vi "BaseProvider_DesignPattern_GetPatterns.vi"(1 "FilterOnProviders(Ignored If Empty)":string, 2 "FilterOnTemplate(Ignored If Empty)":string, 5 "error in (no error)":errorcluster) -> (15 "DesignPatterns":T1[](array[typedef]), 19 "error out":errorcluster)   [LabVIEW 2016]
uses:
  <resource>/Framework/Providers/Open_GDS/ClassProviders/Provider_BaseClassInterface/DesignPatternsData.ctl
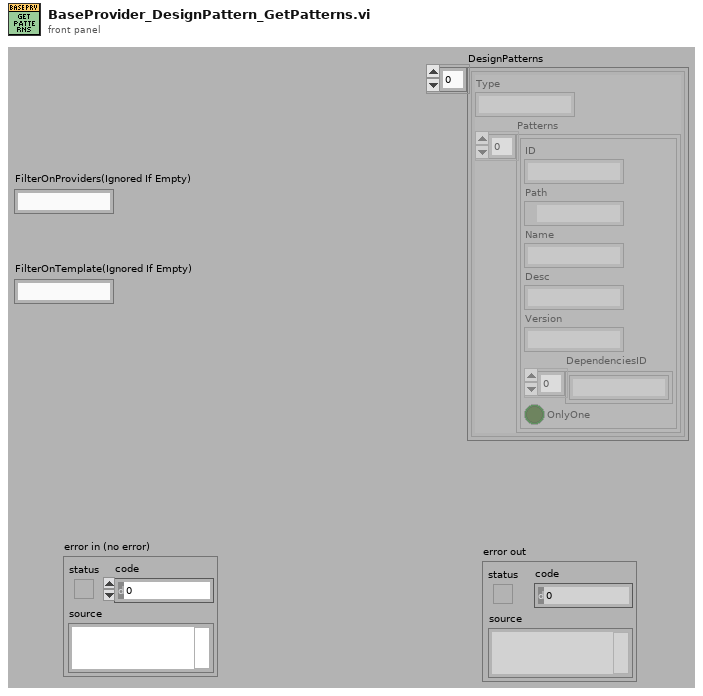
[diagram p1: front panel]
types:
  T1 = typedef "DesignPatternsData.ctl" = cluster{"Type":string, "Patterns":cluster{"ID":string, "Path":path, "Name":string, "Desc":string, "Version":string, "DependenciesID":string[], "OnlyOne":bool}[]}
  T2 = cluster{"Cancelled":bool, "IniFiles":path[], "IniFilesContent":cluster{"ID":string, "Version":string, "PlugIn":path, "Type":string, "Name":string, "Desc":string, "Supports":cluster{"Provider":string, "Templates":string}[], "DependenciesID":string[], "OnlyOne":bool}[], "DesignPatterns":T1[]}
  T3 = cluster{"ID":string, "Version":string, "PlugIn":path, "Type":string, "Name":string, "Desc":string, "Supports":cluster{"Provider":string, "Templates":string}[], "DependenciesID":string[], "OnlyOne":bool}[]
  T4 = cluster{"ID":string, "Version":string, "PlugIn":path, "Type":string, "Name":string, "Desc":string, "Supports":cluster{"Provider":string, "Templates":string}[], "DependenciesID":string[], "OnlyOne":bool}
  T5 = cluster{"ID":string, "Path":path, "Name":string, "Desc":string, "Version":string, "DependenciesID":string[], "OnlyOne":bool}[]
  T6 = cluster{"ID":string, "Path":path, "Name":string, "Desc":string, "Version":string, "DependenciesID":string[], "OnlyOne":bool}
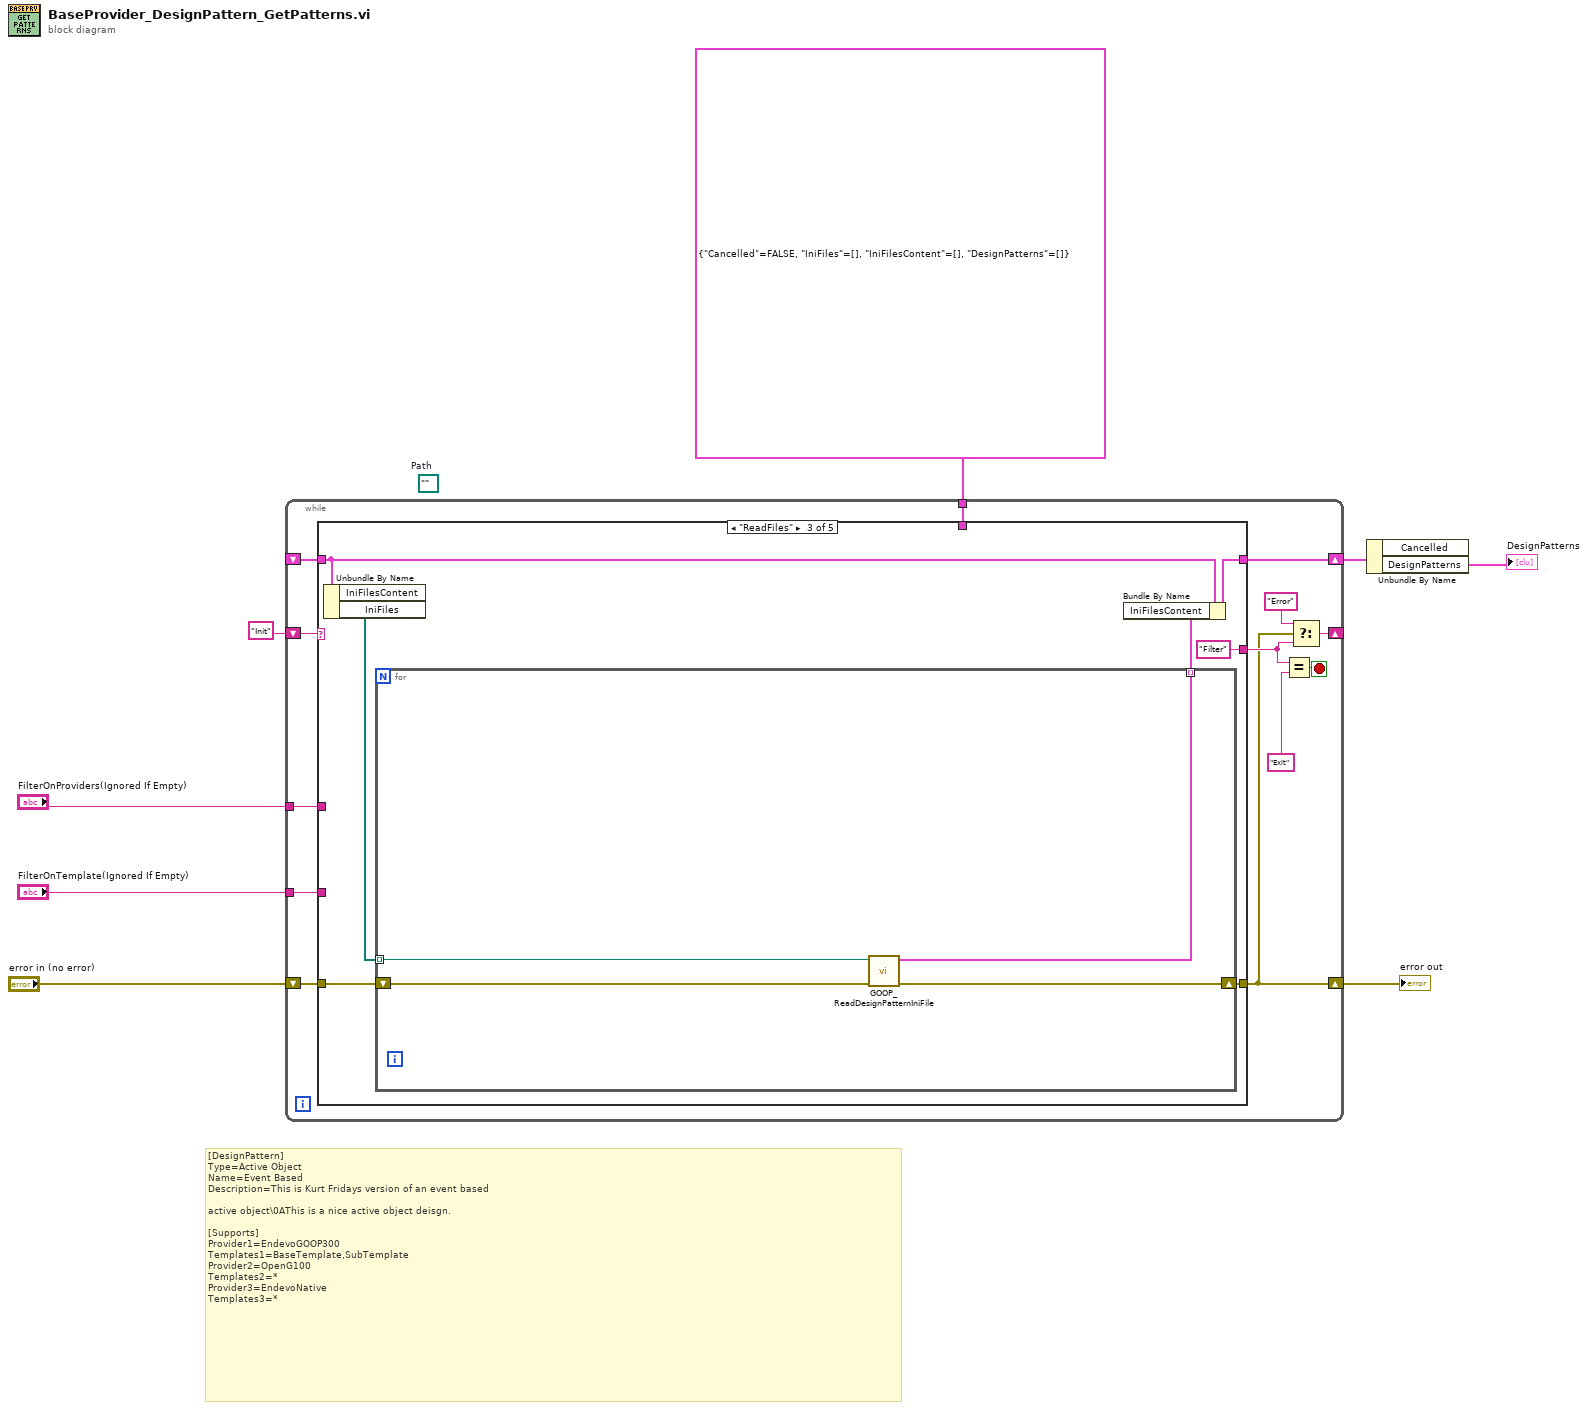
[diagram p0: block diagram]
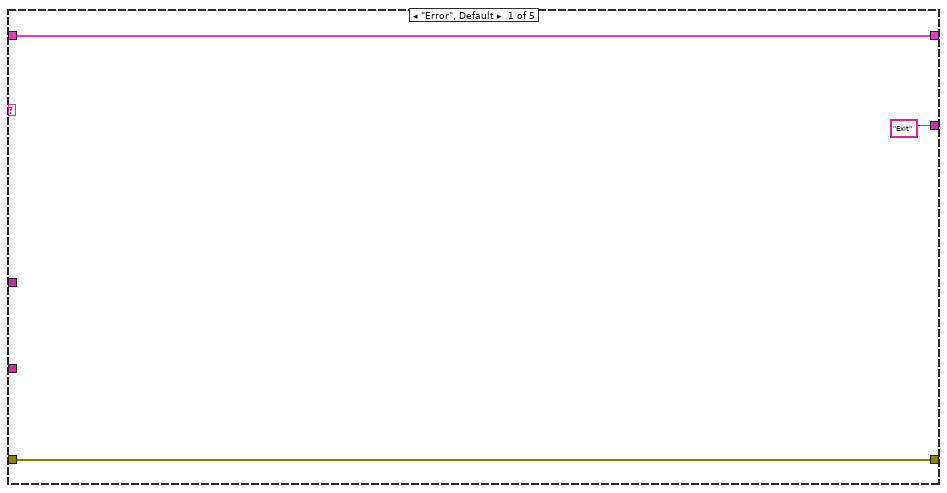
[diagram p2: hidden frame]
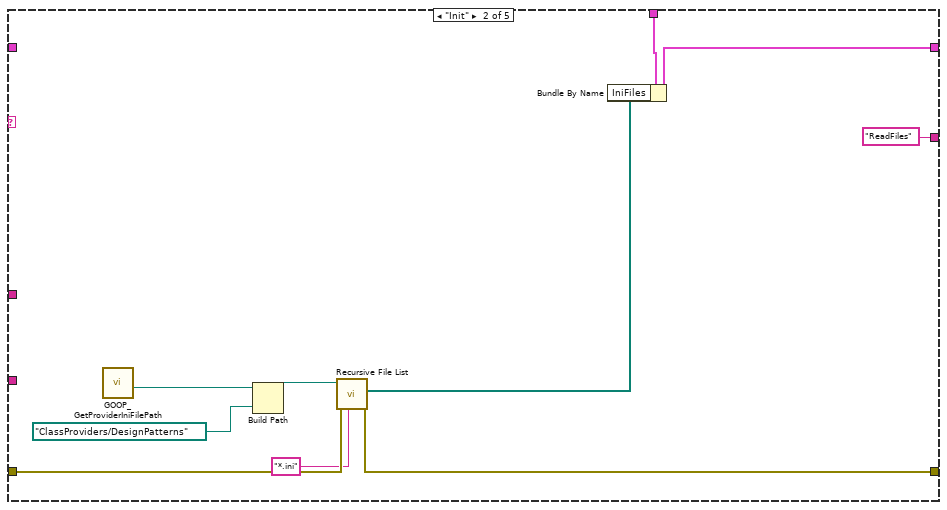
[diagram p3: hidden frame]
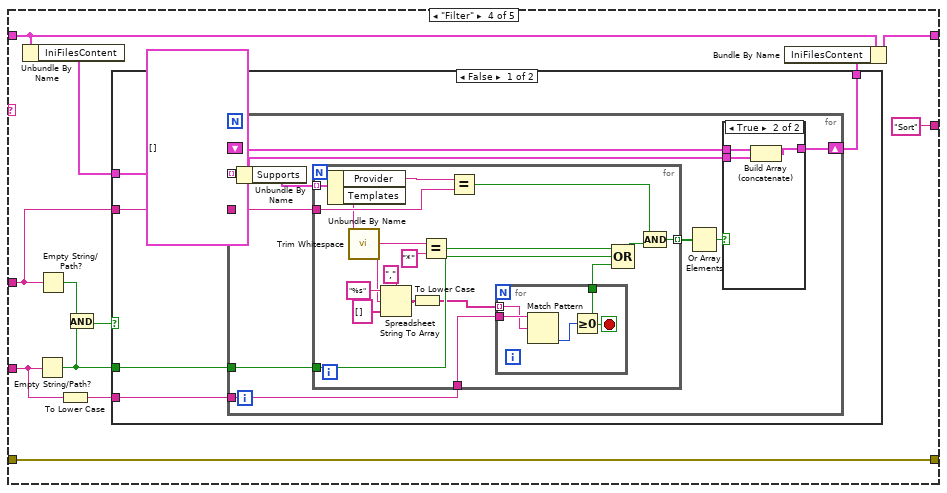
[diagram p4: hidden frame]
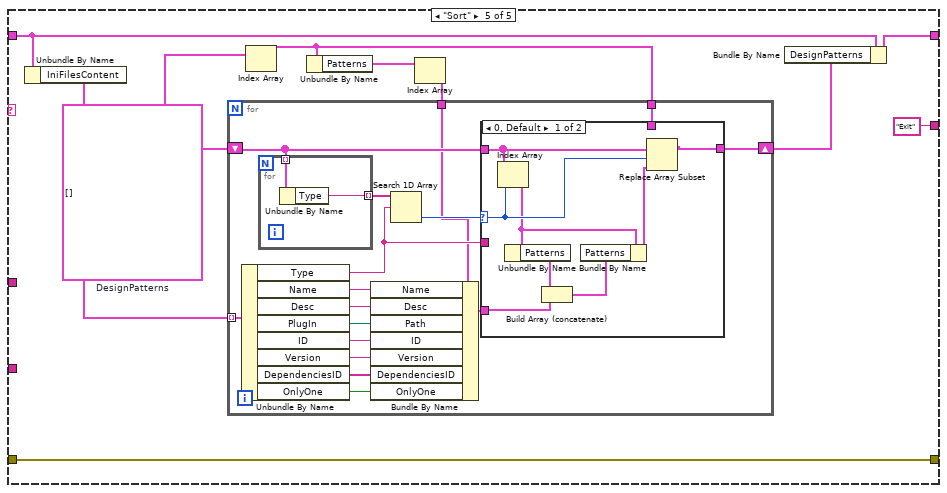
[diagram p7: hidden frame]
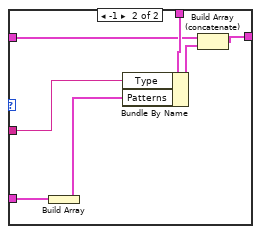
[diagram p8: hidden frame]
diagram:
  (unwired) path ""  # Path
  # "[DesignPattern]\nType=Active Object\nName=Event Based\nDescription=This is Kurt Fridays version of an event based \n\nactive object\\0AThis is a nice active object deisgn.\n\n[Supports]\nProvider1=EndevoGOOP300\nTemplates1=BaseTemplate,SubTemplate\nProvider2=OpenG100\nTemplates2=*\nProvider3=EndevoNative\nTemplates3=*"
  n1 = while {
    shift-right: [w14] -> w5
    shift-left: "error in (no error)" -> [w21]
    shift-right: [w19] -> _
    shift-left: "Init" -> [w20]
    shift-right: [w13] -> w7
    shift-left: _ -> [w12]
    tunnel: "FilterOnProviders(Ignored If Empty)" -> [w11]
    tunnel: "FilterOnTemplate(Ignored If Empty)" -> [w10]
    tunnel: T2 {"Cancelled"=FALSE, "IniFiles"=[], "IniFilesContent"=[], "DesignPatterns"=[]} -> [w9]
    stop <- w18 stop-if-true
    n2 = case shown="\"ReadFiles\"" w20 {
      tunnel: w21 -> [w24 w29 w40 w56 w108]
      tunnel: [w24 w28 w38 w56 w108] -> w14
      tunnel: ["Exit" "ReadFiles" "Filter" "Sort" "Exit"] -> w15
      tunnel: [w22 w33 w36 w51 w106] -> w13
      tunnel: w12 -> [w22 _ w37 w53 w107]
      tunnel: w11 -> [_ _ _ w49 _]
      tunnel: w10 -> [_ _ _ w47 _]
      tunnel: w9 -> [_ w25 _ _ _]
      frame "Error", Default {
      }
      frame "Init" {
        n3 = call <resource>:"GOOP_GetProviderIniFilePath.vi"() -> ("ProviderMainFolder"=w32:path)  [unwired: 10 in, 1 out]
        n4 = Build Path(base path=w32, name or relative path=path "ClassProviders/DesignPatterns" ("base path")) -> (appended path=w30:path)
        n5 = call <vilib>:"Recursive File List.vi"("pattern"="*.ini", "error in (no error)"=w29, "Folder Path"=w30) -> ("error out"=w28:errorcluster, "All Files in Dir"=w26:path[])  [unwired: 4 in, 3 out]
        n6 = Bundle By Name(cluster=w25, "IniFiles"=w26) -> (w33:T2)
      }
      frame "ReadFiles" {
        n7 = Unbundle By Name(w37) -> ("IniFiles"=w39:path[])  [unwired: 1 out]
        n8 = for {
          shift-right: [w44] -> w38
          shift-left: w40 -> [w45]
          tunnel: w39 -> [w42] mode=indexing
          tunnel: [w43] -> w35 mode=indexing
          n9 = call <resource>:"GOOP_ReadDesignPatternIniFile.vi"("error in (no error)"=w45, "Path"=w42) -> ("error out"=w44:errorcluster, "cluster"=w43:T4)  [unwired: 8 in]
        }
        n10 = Bundle By Name(cluster=w37, "IniFilesContent"=w35) -> (w36:T2)
      }
      frame "Filter" {
        n11 = Unbundle By Name(w53) -> ("IniFilesContent"=w57:T3)
        n12 = Empty String/Path?(string/path=w47) -> (empty?=w48:bool)
        n13 = Empty String/Path?(string/path=w49) -> (empty?=w55:bool)
        n14 = To Lower Case(string=w47) -> (all lower case string=w46:string)
        n15 = And(x=w55, y=w48) -> (x .and. y?=w54:bool)
        n16 = case shown="False" w54 {
          tunnel: w57 -> [w63 w99]
          tunnel: [w59 w99] -> w52
          tunnel: w49 -> [w62 _]
          tunnel: w46 -> [w61 _]
          tunnel: w48 -> [w60 _]
          frame False {
            n17 = for {
              tunnel: w63 -> [w65] mode=indexing
              shift-right: [w70] -> w59
              shift-left: T3 [] -> [w71]
              tunnel: w62 -> [w69]
              tunnel: w61 -> [w64]
              tunnel: w60 -> [w68]
              n18 = Unbundle By Name(w65) -> ("Supports"=w72:cluster{"Provider":string, "Templates":string}[])
              n19 = for {
                tunnel: w72 -> [w94] mode=indexing
                tunnel: w69 -> [w92]
                tunnel: w64 -> [w78]
                tunnel: w68 -> [w87]
                tunnel: [w85] -> w67 mode=indexing
                n20 = Unbundle By Name(w94) -> ("Provider"=w93:string, "Templates"=w84:string)
                n21 = call <vilib>:"Trim Whitespace.vi"("string"=w84) -> ("trimmed string"=w83:string)  [unwired: 1 in]
                n22 = Spreadsheet String To Array(delimiter (Tab)=",", format string="%s", spreadsheet string=w83, array type (2D Dbl)=string[] []) -> (array=w88:string[])
                n23 = To Lower Case(string=w88) -> (all lower case string=w79:string[])
                n24 = Equal?(x=w83, y="*" ("element")) -> (x = y?=w80:bool)
                n25 = Equal?(x=w93, y=w92) -> (x = y?=w81:bool)
                n26 = for {
                  tunnel: w79 -> [w95] mode=indexing
                  tunnel: w78 -> [w96]
                  tunnel: [w97] -> w77
                  stop <- w97 stop-if-true
                  n27 = Match Pattern(string=w96, regular expression=w95) -> (offset past match=w98:i32)  [unwired: 1 in, 3 out]
                  n28 = Greater Or Equal To 0?(x=w98) -> (x >= 0?=w97:bool)
                }
                n29 = Compound Arithmetic op=OR(w80, w87, w77) -> (w86:bool)
                n30 = Compound Arithmetic op=AND(w81, w86) -> (w85:bool)
              }
              n31 = Or Array Elements(Boolean array=w67) -> (logical OR=w66:bool)
              n32 = case shown="True" w66 {
                tunnel: w71 -> [w73 w76]
                tunnel: [w73 w75] -> w70
                tunnel: w65 -> [_ w74]
                frame False {
                }
                frame True {
                  n33 = Build Array (concatenate)(w76, w74) -> (w75:T3)
                }
              }
            }
          }
          frame True {
          }
        }
        n34 = Bundle By Name(cluster=w53, "IniFilesContent"=w52) -> (w51:T2)
      }
      frame "Sort" {
        w103 = T1[] []  # DesignPatterns
        n35 = Unbundle By Name(w107) -> ("IniFilesContent"=w109:T3)
        n36 = Index Array(array=w103) -> (element=w102:T1)  [unwired: 1 in]
        n37 = Unbundle By Name(w102) -> ("Patterns"=w101:T5)
        n38 = Index Array(array=w101) -> (element=w100:T6)  [unwired: 1 in]
        n39 = for {
          tunnel: w109 -> [w124] mode=indexing
          shift-right: [w125] -> w104
          shift-left: w103 -> [w123]
          tunnel: w102 -> [w120]
          tunnel: w100 -> [w115]
          n40 = Unbundle By Name(w124) -> ("Type"=w119:string, "Name"=w118:string, "Desc"=w117:string, "PlugIn"=w116:path, "ID"=w113:string, "Version"=w112:string, "DependenciesID"=w111:string[], "OnlyOne"=w110:bool)
          n41 = for {
            tunnel: w123 -> [w127] mode=indexing
            tunnel: [w126] -> w122 mode=indexing
            n42 = Unbundle By Name(w127) -> ("Type"=w126:string)
          }
          n43 = Bundle By Name(cluster=w115, "Name"=w118, "Desc"=w117, "Path"=w116, "ID"=w113, "Version"=w112, "DependenciesID"=w111, "OnlyOne"=w110) -> (w114:T6)
          n44 = Search 1D Array(1D array=w122, element=w119) -> (index of element=w121:i32)  [unwired: 1 in]
          n45 = case shown="0, Default" w121 {
            selector: w121 -> [w134 _]
            tunnel: w123 -> [w135 w136]
            tunnel: [w128 w142] -> w125
            tunnel: w120 -> [_ w141]
            tunnel: w119 -> [_ w137]
            tunnel: w114 -> [w131 w138]
            frame 0, Default {
              n46 = Index Array(array=w135, index=w134) -> (element=w133:T1)
              n47 = Unbundle By Name(w133) -> ("Patterns"=w132:T5)
              n48 = Build Array (concatenate)(w132, w131) -> (w130:T5)
              n49 = Bundle By Name(cluster=w133, "Patterns"=w130) -> (w129:T1)
              n50 = Replace Array Subset(array=w135, new element=w129, index=w134) -> (w128:T1[])
            }
            frame -1 {
              n51 = Build Array(w138) -> (w139:T5)
              n52 = Bundle By Name(cluster=w141, "Type"=w137, "Patterns"=w139) -> (w140:T1)
              n53 = Build Array (concatenate)(w136, w140) -> (w142:T1[])
            }
          }
        }
        n54 = Bundle By Name(cluster=w107, "DesignPatterns"=w104) -> (w106:T2)
      }
    }
    n55 = Equal?(x=w15, y="Exit") -> (x = y?=w18:bool)
    n56 = Select(t="Error", s=w14, f=w15) -> (s? t:f=w19:string)
  }
  "error out" <- w5
  n57 = Unbundle By Name(w7) -> ("DesignPatterns"=→"DesignPatterns":T1[])  [unwired: 1 out]
